vi "Save Table Test_For 工單號碼.vi"(8 "error in (no error)":errorcluster, 11 "工單號碼":string) -> (0 "error out":errorcluster, 3 "條碼的Index":i32)   [LabVIEW 2019]
uses:
  Ctrl/Table Save.ctl
  LLB/Message/Ctrl/LogType.ctl
  <vilib>/Utility/sysdir.llb/System Directory Type.ctl
  <vilib>/Utility/file.llb/Write Delimited Spreadsheet (string).vi
  LLB/Message/MsgShowAndLog.lvlib
panel:
  out "Read SN Table":string[][](array[string])
  in  "Base Path":path=path "D:/Vicomm"
  out "element":string
  in  "Cluster":cluster{"Table Control":string[][]}={"Table Control"=[["PCBA BARCODE", ""], ["硬體(Tool初始化)", ""], ["company(Tool初始化)", ""], ["耗電流 uA(電流表)", "T"], ["電池負載電壓", "T"], ["晶片ID(Tool FORMAT)", "F"], ["雷雕ID(TOOl scan、藍芽接收器)", "S"], ["Format(Tool FORMAT)", "F"], ["Programe(Tool Programe)", "P"]]}
  # "-1 : 未找到條碼"
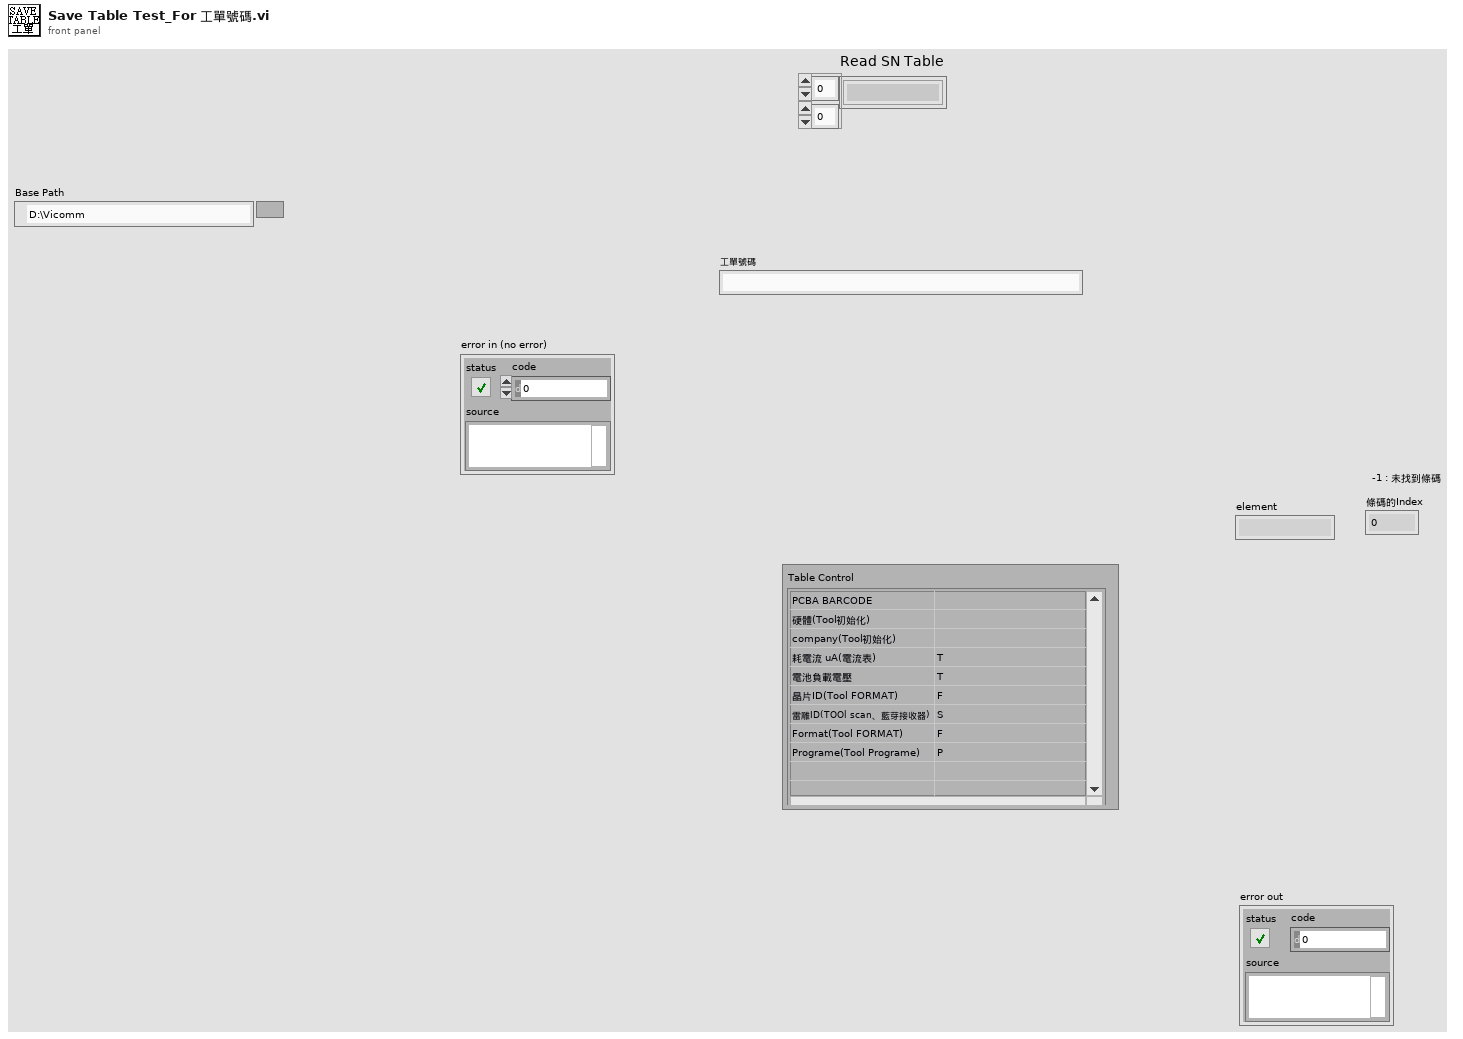
[diagram p1: front panel]
types:
  T1 = typedef "Table Save.ctl" = enum16{"initial", "Add", "Write", "Replace", "Delete", "REad", "RedTable", "Load"}
  T2 = enum16{"open", "replace", "create", "open or create", "replace or create", "replace or create with confirmation"}
  T3 = typedef "MsgShowAndLog.lvlib/LogType.ctl" = enum16{"Auto", "Manual", "Handshake", "Error"}
  T4 = typedef "System Directory Type.ctl" = i32
  T5 = typedef "LVDateTimeRec.ctl" = cluster{"fractional second":dbl, "second":i32, "minute":i32, "hour":i32, "day of month":i32, "month":i32, "year":i32, "day of week":i32, "day of year":i32, "DST":i32}
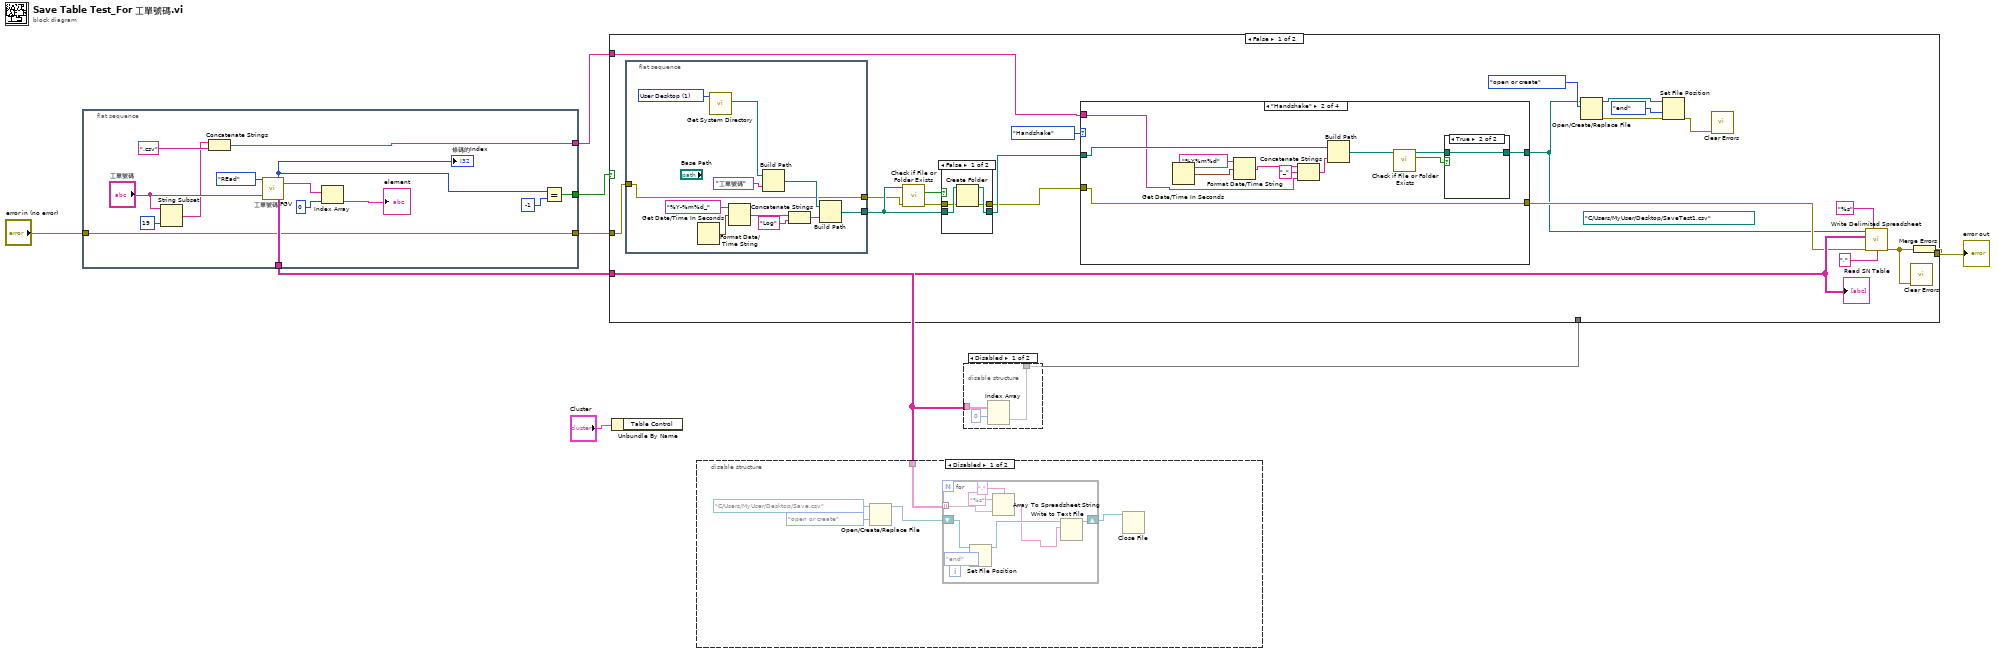
[diagram p0: block diagram]
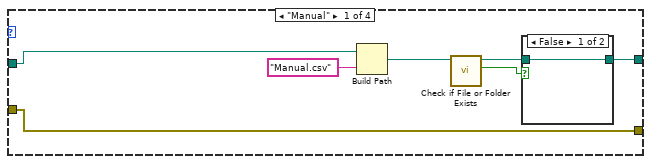
[diagram p2: hidden frame]
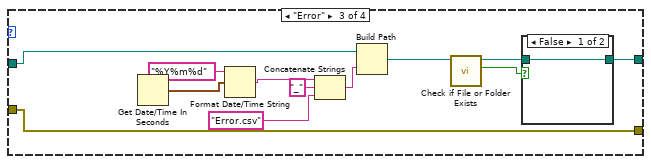
[diagram p5: hidden frame]
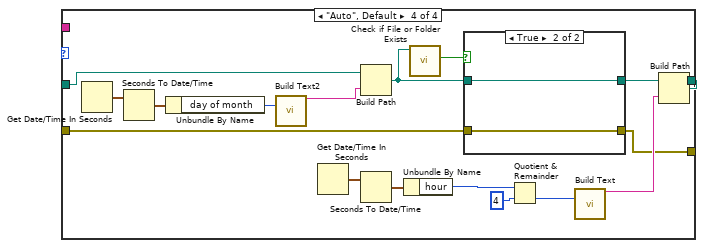
[diagram p7: hidden frame]
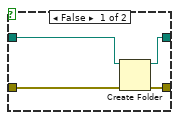
[diagram p8: hidden frame]
diagram:
  n1 = flat-sequence {
    tunnel: [w22] -> w1
    tunnel: [w16] -> w6
    tunnel: "error in (no error)" -> [w13]
    tunnel: [w13] -> w3
    tunnel: [w12] -> w4
    frame #0 {
      n2 = String Subset(string="工單號碼", length (rest)=19 ("length (rest)")) -> (substring=w10:string)  [unwired: 1 in]
      n3 = Concatenate Strings(w10, ".csv") -> (w22:string)
      n4 = call "工單號碼 FGV.vi"("Action"=Table_Save."REad", "工單號碼"="工單號碼") -> ("工單號碼的Index"=w15:i32, "Read SN Table"=w16:string[][], "Barcode Array"=w18:string[])  [unwired: 10 in, 5 out]
      "條碼的Index" <- w15
      n5 = Index Array(array=w18, index=0) -> (element=→"element":string)
      n6 = Equal?(x=w15, y=-1) -> (x = y?=w12:bool)
    }
  }
  n7 = Unbundle By Name("Cluster") -> ()  [unwired: 1 out]
  n8 = disable-structure shown="Disabled" {
    disable-tunnel: w6 -> [w23 _]
    frame Disabled {
      n9 = Open/Create/Replace File(file path (use dialog)=path "C:/Users/MyUser/Desktop/Save.csv", operation (0:open)=T2."open or create") -> (refnum out=w27:refnum<file>)  [unwired: 4 in, 2 out]
      n10 = for {
        tunnel: w23 -> [w35] mode=indexing
        shift-right: [w32] -> w25
        shift-left: w27 -> [w31]
        n11 = Set File Position(refnum=w31, from (0:start)=enum16{"start", "end", "current"}."end") -> (refnum out=w30:refnum<file>)  [unwired: 2 in, 1 out]
        n12 = Array To Spreadsheet String(delimiter (Tab)=",", array=w35, 3:"%s" ("format string")) -> (spreadsheet string=w28:string)
        n13 = Write to Text File(file (use dialog)=w30, text=w28) -> (refnum out=w32:refnum<file>)  [unwired: 2 in, 2 out]
      }
      n14 = Close File(refnum=w25) -> ()  [unwired: 1 in, 2 out]
    }
    frame Enabled {
    }
  }
  n15 = disable-structure shown="Disabled" {
    disable-tunnel: [w37 _] -> w8
    disable-tunnel: w6 -> [w36 _]
    frame Disabled {
      n16 = Index Array(array=w36, index (row)=0) -> (element=w37:string[])  [unwired: 1 in]
    }
    frame Enabled {
    }
  }
  n17 = case shown="False" w4 {
    tunnel: w8 -> [_ _]
    tunnel: w6 -> [w48 _]
    tunnel: w3 -> [w42 w137]
    tunnel: [w41 w137] -> w2
    tunnel: w1 -> [w40 _]
    frame False {
      (unwired) path "C:/Users/MyUser/Desktop/SaveTest1.csv" ("file path (dialog if empty)")
      n18 = flat-sequence {
        tunnel: [w123] -> w58
        tunnel: w42 -> [w122]
        tunnel: [w122] -> w56
        frame #0 {
          w121 = T4 1 items=["User Home"=0, "User Desktop"=1, "User Documents"=2, "User Application Data"=3, "User Preferences"=4, "User Temporary"=5, "Public Documents"=6, "Public Application Data"=7, "Public Preferences"=8, "Public Cache"=13, "System Core Libraries"=9, "System Installed Libraries"=10, "Application Files"=11, "Boot Volume Root"=12] ("system directory type")
          n19 = Get Date/Time In Seconds() -> (seconds since 1Jan1904=w124:timestamp)
          n20 = call <vilib>:"Get System Directory.vi"("system directory type"=w121) -> ("system directory"=w120:path)  [unwired: 10 in]
          n21 = Format Date/Time String(time format string (%c)="%Y-%m%d_", seconds (now)=w124) -> (date/time string=w126:string)  [unwired: 1 in]
          n22 = Build Path(base path=w120, name or relative path="工單號碼") -> (appended path=w130:path)
          n23 = Concatenate Strings(w126, "Log") -> (w128:string)
          n24 = Build Path(base path=w130, name or relative path=w128) -> (appended path=w123:path)
        }
      }
      n25 = call <vilib>:"Check if File or Folder Exists.vi"("error in (no error)"=w56, "path"=w58) -> ("error out"=w59:errorcluster, "file or folder exists?"=w57:bool)  [unwired: 7 in, 1 out]
      n26 = case shown="False" w57 {
        tunnel: w58 -> [w134 w136]
        tunnel: [w133 w136] -> w54
        tunnel: w59 -> [w132 w135]
        tunnel: [w131 w135] -> w53
        frame False {
          n27 = Create Folder(path (use dialog)=w134, error in=w132) -> (created path=w133:path, error out=w131:errorcluster)  [unwired: 1 in, 1 out]
        }
        frame True {
        }
      }
      n28 = case shown="\"Handshake\"" LogType."Handshake" ("LogType") {
        tunnel: w54 -> [w66 w80 w94 w108]
        tunnel: w53 -> [w60 w75 w89 w101]
        tunnel: [w61 w76 w90 w100] -> w39
        tunnel: [w60 w75 w89 w97] -> w43
        tunnel: w40 -> [_ w69 _ _]
        frame "Manual" {
          n29 = Build Path(base path=w66, name or relative path="Manual.csv") -> (appended path=w64:path)
          n30 = call <vilib>:"Check if File or Folder Exists.vi"("path"=w64) -> ("file or folder exists?"=w63:bool, "dup path"=w62:path)  [unwired: 8 in, 1 out]
          n31 = case shown="False" w63 {
            tunnel: w62 -> [w67 w68]
            tunnel: [w67 w68] -> w61
            frame False {
            }
            frame True {
            }
          }
        }
        frame "Handshake" {
          n32 = Get Date/Time In Seconds() -> (seconds since 1Jan1904=w74:timestamp)
          n33 = Format Date/Time String(time format string (%c)="%Y%m%d", seconds (now)=w74) -> (date/time string=w71:string)  [unwired: 1 in]
          n34 = Concatenate Strings(w71, "_" ("string"), w69) -> (w72:string)
          n35 = Build Path(base path=w80, name or relative path=w72) -> (appended path=w79:path)
          n36 = call <vilib>:"Check if File or Folder Exists.vi"("path"=w79) -> ("file or folder exists?"=w78:bool, "dup path"=w77:path)  [unwired: 8 in, 1 out]
          n37 = case shown="True" w78 {
            tunnel: w77 -> [w81 w82]
            tunnel: [w81 w82] -> w76
            frame False {
            }
            frame True {
            }
          }
        }
        frame "Error" {
          n38 = Get Date/Time In Seconds() -> (seconds since 1Jan1904=w88:timestamp)
          n39 = Format Date/Time String(time format string (%c)="%Y%m%d", seconds (now)=w88) -> (date/time string=w84:string)  [unwired: 1 in]
          n40 = Concatenate Strings(w84, "_" ("string"), "Error.csv" ("name or relative path")) -> (w86:string)
          n41 = Build Path(base path=w94, name or relative path=w86) -> (appended path=w93:path)
          n42 = call <vilib>:"Check if File or Folder Exists.vi"("path"=w93) -> ("file or folder exists?"=w92:bool, "dup path"=w91:path)  [unwired: 8 in, 1 out]
          n43 = case shown="False" w92 {
            tunnel: w91 -> [w95 w96]
            tunnel: [w95 w96] -> w90
            frame False {
            }
            frame True {
            }
          }
        }
        frame "Auto", Default {
          n44 = Get Date/Time In Seconds() -> (seconds since 1Jan1904=w106:timestamp)
          n45 = Seconds To Date/Time(time stamp (now)=w106) -> (date time rec=w105:T5)  [unwired: 1 in]
          n46 = Unbundle By Name(w105) -> ("day of month"=w107:i32)
          n47 = call "Build Text2"("Date"=w107) -> ("Result"=w104:string)  [unwired: 13 in, 1 out]
          n48 = Get Date/Time In Seconds() -> (seconds since 1Jan1904=w113:timestamp)
          n49 = Build Path(base path=w108, name or relative path=w104) -> (appended path=w99:path)
          n50 = Seconds To Date/Time(time stamp (now)=w113) -> (date time rec=w112:T5)  [unwired: 1 in]
          n51 = Unbundle By Name(w112) -> ("hour"=w110:i32)
          n52 = call <vilib>:"Check if File or Folder Exists.vi"("path"=w99) -> ("file or folder exists?"=w98:bool)  [unwired: 8 in, 2 out]
          n53 = case shown="True" w98 {
            tunnel: w99 -> [w117 w119]
            tunnel: [w116 w119] -> w103
            tunnel: w101 -> [w115 w118]
            tunnel: [w114 w118] -> w97
            frame False {
              n54 = Create Folder(path (use dialog)=w117, error in=w115) -> (created path=w116:path, error out=w114:errorcluster)  [unwired: 1 in, 1 out]
            }
            frame True {
            }
          }
          n55 = Quotient & Remainder(x=w110, y=4) -> (floor(x/y)=w109:i32)  [unwired: 1 out]
          n56 = call "Build Text"("Time"=w109) -> ("Result"=w102:string)  [unwired: 13 in, 1 out]
          n57 = Build Path(base path=w103, name or relative path=w102) -> (appended path=w100:path)
        }
      }
      n58 = Open/Create/Replace File(file path (use dialog)=w39, operation (0:open)=T2."open or create") -> (refnum out=w50:refnum<file>, error out=w52:errorcluster)  [unwired: 4 in, 1 out]
      n59 = Set File Position(refnum=w50, from (0:start)=enum16{"start", "end", "current"}."end", error in=w52) -> (error out=w47:errorcluster)  [unwired: 1 in, 1 out]
      n60 = call <vilib>:"Clear Errors.vi"("error in (no error)"=w47) -> ()  [unwired: 5 in, 2 out]
      n61 = call-poly <vilib>:"Write Delimited Spreadsheet.vi"("file path (dialog if empty)"=w39, "format (%s)"="%s", "2D data"=w48, "error in (no error)"=w43, "delimiter (\\t)"="," ("delimiter (\\t)")) -> ("error out"=w44:errorcluster)  [unwired: 9 in, 1 out]
      n62 = call <vilib>:"Clear Errors.vi"("error in (no error)"=w44) -> ()  [unwired: 5 in, 2 out]
      n63 = Merge Errors(w44) -> (w41:errorcluster)
      "Read SN Table" <- w48
    }
    frame True {
    }
  }
  "error out" <- w2
